vi "Append Image to Report (string).vi"(0 "report in":refnum<class "NI_HTML.lvclass">, 1 "alignment (default)":T1, 2 "MS Office parameters":T2, 7 "path or URL of image":string, 9 "caption or alternative string":string, 11 "error in (no error)":errorcluster) -> (4 "report out":refnum<class "NI_HTML.lvclass">, 8 "start out (Word)":i32, 10 "end out (Word)":i32, 15 "error out":errorcluster)   [LabVIEW 2015, in "NI_HTML.lvclass"]
doc: "For an HTML report, the VI embeds a link to an image into the report. For a standard report, the VI appends the image from a file. You can wire either a path to the image or a string that contains the image URL to this polymorphic VI. The data type you wire to the <B>path or URL of image</B> input determines the polymorphic instance to use."
uses:
  <vilib>/Utility/NIReport.llb/HTML/NI_HTML.lvclass
  <vilib>/Utility/NIReport.llb/HTML Report Image Alignment.ctl
  <vilib>/Utility/NIReport.llb/HTML/NI_HTML.lvclass/NI_HTML.ctl
  <vilib>/Utility/NIReport.llb/NI_ReportGenerationCore.lvlib
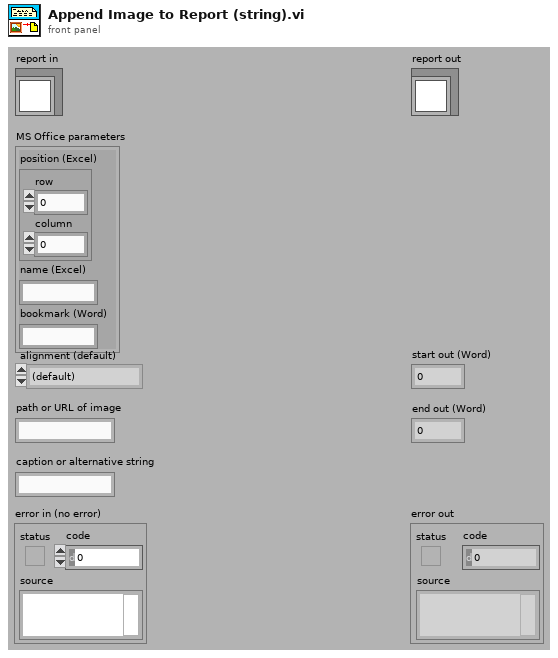
[diagram p1: front panel]
types:
  T1 = typedef "NI_ReportGenerationCore.lvlib/HTML Report Image Alignment.ctl" = enum16{"(default)", "LEFT", "RIGHT", "TOP", "TEXTTOP", "MIDDLE", "ABSMIDDLE", "BASELINE", "BOTTOM", "ABSBOTTOM"}
  T2 = cluster{"position (Excel)":cluster{"row":i32, "column":i32}, "name (Excel)":string, "bookmark (Word)":string}
  T3 = typedef "NI_ReportGenerationCore.lvlib/HTML Report Data.ctl" = cluster{"Body Text":string, "Font Tag":string, "Title Text":string, "Header Text":string, "Footer Text":string, "Image List":path[]}
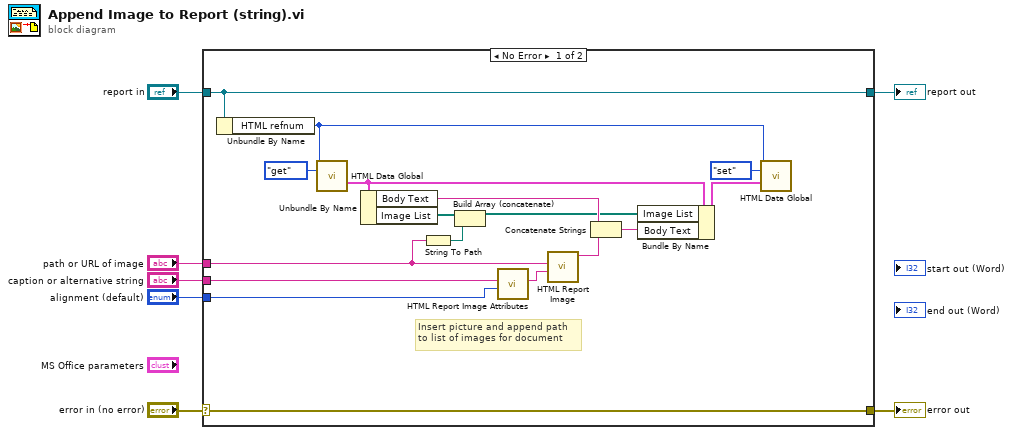
[diagram p0: block diagram]
diagram:
  n1 = case shown="No Error" "error in (no error)" {
    selector: "error in (no error)" -> [w24 w26]
    tunnel: [w24 w26] -> w6
    tunnel: [w14 w25] -> w4
    tunnel: "report in" -> [w14 w25]
    tunnel: "caption or alternative string" -> [w19 _]
    tunnel: "path or URL of image" -> [w18 _]
    tunnel: "alignment (default)" -> [w17 _]
    frame No Error {
      # "Insert picture and append path\nto list of images for document"
      n2 = Unbundle By Name(w14) -> ("HTML refnum"=w8:u32)
      n3 = call <vilib>:"HTML Data Global.vi"("HTML refnum"=w8, "menu"=enum16{"init", "get", "set", "delete"}."get") -> ("HTML report data out"=w12:T3)  [unwired: 1 in, 12 out]
      n4 = Unbundle By Name(w12) -> ("Body Text"=w13:string, "Image List"=w16:path[])
      n5 = String To Path(string=w18) -> (path=w22:path)
      n6 = Build Array (concatenate)(w16, w22) -> (w11:path[])
      n7 = call <vilib>:"HTML Report Image Attributes.vi"("alignment (default)"=w17, "alt - alternative string"=w19) -> ("attributes out"=w20:string)  [unwired: 5 out]
      n8 = call <vilib>:"HTML Report Image.vi"("image attributes"=w20, "src - URL of image to embed"=w18) -> ("HTML out"=w21:string)  [unwired: 2 in, 7 out]
      n9 = Concatenate Strings(w13, w21) -> (w23:string)
      n10 = Bundle By Name(cluster=w12, "Image List"=w11, "Body Text"=w23) -> (w9:T3)
      n11 = call <vilib>:"HTML Data Global.vi"("HTML refnum"=w8, "menu"=enum16{"init", "get", "set", "delete"}."set", "HTML report data in"=w9) -> ()  [unwired: 13 out]
    }
    frame Error {
    }
  }
  "error out" <- w6
  "report out" <- w4
